vi "ConvertTimeStampToHHMMSS.vi"(11 "Timestamp":dbl) -> (3 "HH:MM:SS":string)   [LabVIEW 2014]
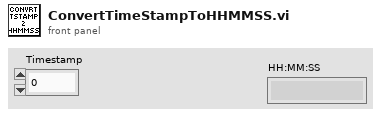
[diagram p1: front panel]
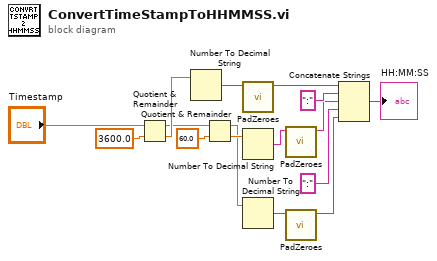
[diagram p0: block diagram]
diagram:
  n1 = Quotient & Remainder(x="Timestamp", y=3600.0) -> (x-y*floor(x/y)=w11:dbl, floor(x/y)=w14:dbl)
  n2 = Number To Decimal String(number=w14) -> (decimal integer string=w6:string)  [unwired: 1 in]
  n3 = Quotient & Remainder(x=w11, y=60.0) -> (x-y*floor(x/y)=w8:dbl, floor(x/y)=w10:dbl)
  n4 = call "PadZeroes.vi"("String"=w6) -> ("Padded String"=w5:string)  [unwired: 10 in]
  n5 = Number To Decimal String(number=w10) -> (decimal integer string=w4:string)  [unwired: 1 in]
  n6 = Number To Decimal String(number=w8) -> (decimal integer string=w2:string)  [unwired: 1 in]
  n7 = call "PadZeroes.vi"("String"=w4) -> ("Padded String"=w3:string)  [unwired: 10 in]
  n8 = call "PadZeroes.vi"("String"=w2) -> ("Padded String"=w1:string)  [unwired: 10 in]
  n9 = Concatenate Strings(w5, ":" ("string"), w3, ":" ("string"), w1) -> (→"HH:MM:SS":string)
